vi "daemon.vi"(8 "error in (no error)":errorcluster, 11 "ComicVine_manager.lvclass":refnum<class "ComicVine_manager.lvclass">) -> ()   [LabVIEW 2024, in "ComicVine_manager.lvclass"]
uses:
  ComicVine_manager.lvclass
  ComicVine_manager.lvclass/ComicVine_manager.ctl
  states--enum.ctl
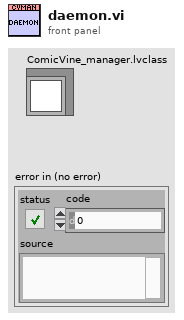
[diagram p1: front panel]
types:
  T1 = typedef "ComicVine_manager.lvclass/states--enum.ctl" = enum16{"start", "running", "start timer", "update file", "set directories", "wait", "shutdown"}
  T2 = cluster{"volume directory":path, "issue directory":path}
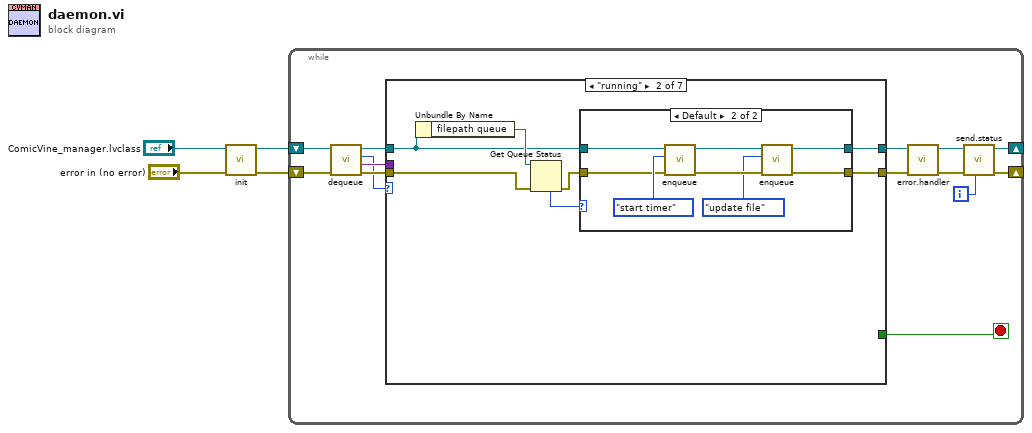
[diagram p0: block diagram]
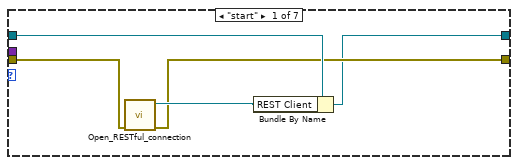
[diagram p2: hidden frame]
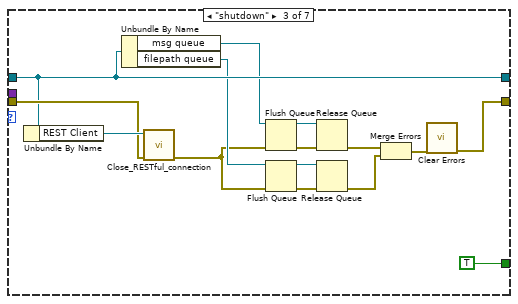
[diagram p4: hidden frame]
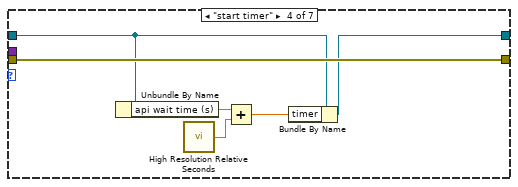
[diagram p5: hidden frame]
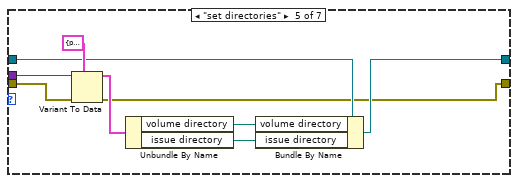
[diagram p6: hidden frame]
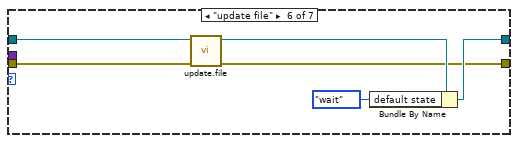
[diagram p7: hidden frame]
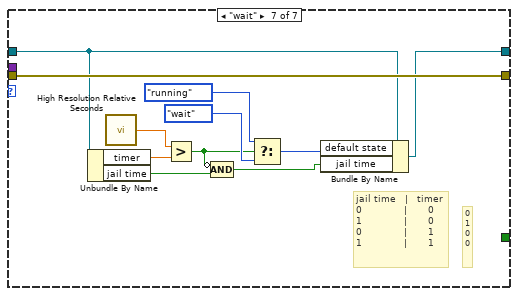
[diagram p8: hidden frame]
diagram:
  n1 = call "init.vi"("error in (no error)"="error in (no error)", "ComicVine_manager in"="ComicVine_manager.lvclass") -> ("error out"=w1:errorcluster, "ComicVine_manager out"=w3:refnum<class "ComicVine_manager.lvclass">)  [unwired: 8 in]
  n2 = while {
    shift-right: [w10] -> _
    shift-left: w3 -> [w18]
    shift-right: [w9] -> _
    shift-left: w1 -> [w17]
    i -> [w11]
    stop <- w12 stop-if-true
    n3 = call "dequeue.vi"("error in (no error)"=w17, "ComicVine_manager in"=w18) -> ("error out"=w16:errorcluster, "data"=w15:variant, "cmd"=w13:T1, "ComicVine_manager out"=w14:refnum<class "ComicVine_manager.lvclass">)  [unwired: 6 in]
    n4 = case shown="\"running\"" w13 {
      tunnel: w16 -> [w20 w29 w53 w61 w68 w71 w87]
      tunnel: w15 -> [_ _ _ _ w69 _ _]
      tunnel: w14 -> [w23 w27 w52 w58 w66 w73 w84]
      tunnel: [w19 w24 w52 w56 w63 w75 w80] -> w8
      tunnel: [w21 w25 w41 w61 w62 w72 w87] -> w7
      tunnel: [_ _ TRUE _ _ _ _] -> w12
      frame "start" {
        n5 = call "Open_RESTful_connection.vi"("error in (no error)"=w20) -> ("error out"=w21:errorcluster, "REST Client out"=w22:refnum<class "REST Client.lvclass">)  [unwired: 9 in]
        n6 = Bundle By Name(cluster=w23, "REST Client"=w22) -> (w19:refnum<class "ComicVine_manager.lvclass">)
      }
      frame "running" {
        n7 = Unbundle By Name(w27) -> ("filepath queue"=w30:refnum<queue>)
        n8 = Get Queue Status(queue=w30, error in (no error)=w29) -> (error out=w26:errorcluster, # elements in queue=w28:i32)  [unwired: 1 in, 6 out]
        n9 = case shown="Default" w28 {
          tunnel: w27 -> [w31 w40]
          tunnel: w26 -> [w32 w38]
          tunnel: [w32 w36] -> w25
          tunnel: [w31 w34] -> w24
          frame 0 {
          }
          frame Default {
            n10 = call "enqueue.vi"("error in (no error)"=w38, "cmd"=states--enum."start timer" ("default state"), "ComicVine_manager in"=w40) -> ("error out"=w37:errorcluster, "ComicVine_manager out"=w35:refnum<class "ComicVine_manager.lvclass">)  [unwired: 7 in]
            n11 = call "enqueue.vi"("error in (no error)"=w37, "cmd"=states--enum."update file" ("default state"), "ComicVine_manager in"=w35) -> ("error out"=w36:errorcluster, "ComicVine_manager out"=w34:refnum<class "ComicVine_manager.lvclass">)  [unwired: 7 in]
          }
        }
      }
      frame "shutdown" {
        n12 = Unbundle By Name(w52) -> ("REST Client"=w54:refnum<class "REST Client.lvclass">)
        n13 = Unbundle By Name(w52) -> ("msg queue"=w49:refnum<queue>, "filepath queue"=w51:refnum<queue>)
        n14 = call "Close_RESTful_connection.vi"("error in (no error)"=w53, "REST Client in"=w54) -> ("error out"=w47:errorcluster)  [unwired: 9 in]
        n15 = Flush Queue(queue=w49, error in (no error)=w47) -> (queue out=w48:refnum<queue>, error out=w46:errorcluster)  [unwired: 1 out]
        n16 = Flush Queue(queue=w51, error in (no error)=w47) -> (queue out=w50:refnum<queue>, error out=w43:errorcluster)  [unwired: 1 out]
        n17 = Release Queue(queue=w48, error in (no error)=w46) -> (error out=w45:errorcluster)  [unwired: 1 in, 2 out]
        n18 = Release Queue(queue=w50, error in (no error)=w43) -> (error out=w44:errorcluster)  [unwired: 1 in, 2 out]
        n19 = Merge Errors(w45, w44) -> (w42:errorcluster)
        n20 = call <vilib>:"Clear Errors.vi"("error in (no error)"=w42) -> ("error out"=w41:errorcluster)  [unwired: 5 in, 1 out]
      }
      frame "start timer" {
        n21 = Unbundle By Name(w58) -> ("api wait time (s)"=w60:dbl)
        n22 = call <vilib>:"High Resolution Relative Seconds.vi"() -> ("relative seconds"=w59:dbl)
        n23 = Add(x=w60, y=w59) -> (x+y=w57:dbl)
        n24 = Bundle By Name(cluster=w58, "timer"=w57) -> (w56:refnum<class "ComicVine_manager.lvclass">)
      }
      frame "set directories" {
        n25 = Variant To Data(error in=w68, type=T2 {"volume directory"=path "", "issue directory"=path ""}, Variant=w69) -> (data=w67:T2, error out=w62:errorcluster)
        n26 = Unbundle By Name(w67) -> ("volume directory"=w65:path, "issue directory"=w64:path)
        n27 = Bundle By Name(cluster=w66, "volume directory"=w65, "issue directory"=w64) -> (w63:refnum<class "ComicVine_manager.lvclass">)
      }
      frame "update file" {
        n28 = call "update.file.vi"("error in (no error)"=w71, "ComicVine_manager in"=w73) -> ("error out"=w72:errorcluster, "ComicVine_manager out"=w74:refnum<class "ComicVine_manager.lvclass">)  [unwired: 8 in]
        n29 = Bundle By Name(cluster=w74, "default state"=states--enum."wait") -> (w75:refnum<class "ComicVine_manager.lvclass">)
      }
      frame "wait" {
        # "0\n1\n0\n0"
        # "jail time   |   timer\n0              |       0\n1              |       0\n0              |       1\n1              |       1"
        n30 = Unbundle By Name(w84) -> ("timer"=w86:dbl, "jail time"=w77:bool)
        n31 = call <vilib>:"High Resolution Relative Seconds.vi"() -> ("relative seconds"=w85:dbl)
        n32 = Greater?(x=w85, y=w86) -> (0:w78:bool)
        n33 = Compound Arithmetic op=AND(invert w78, w77) -> (w79:bool)
        n34 = Select(t=states--enum."running" ("default state"), s=w78, f=states--enum."wait") -> (s? t:f=w81:T1)
        n35 = Bundle By Name(cluster=w84, "default state"=w81, "jail time"=w79) -> (w80:refnum<class "ComicVine_manager.lvclass">)
      }
    }
    n36 = call "error.handler.vi"("error in (no error)"=w7, "ComicVine_manager in"=w8) -> ("error out"=w6:errorcluster, "ComicVine_manager out"=w5:refnum<class "ComicVine_manager.lvclass">)  [unwired: 8 in]
    n37 = call "send.status.vi"("iteration"=w11, "error in (no error)"=w6, "ComicVine_manager in"=w5) -> ("error out"=w9:errorcluster, "ComicVine_manager out"=w10:refnum<class "ComicVine_manager.lvclass">)  [unwired: 7 in]
  }
